vi "CalcDialogPanelBounds.vi"(8 "error in (no error)":errorcluster, 9 "Height":i32, 10 "Width":i32, 11 "Montior":i32) -> (0 "error out":errorcluster, 3 "Front Panel Window:Panel Bounds":T1)   [LabVIEW 2018, in "LcWebView.lvclass"]
doc: "This utility will fit (resize and center) a VI (defined by the \"VI Ref\" input) about the all of the Front Panel object. It will add a border defined by border spacing in units of pixels. If no VI Reference is passed in, it will operate on the calling VI."
uses:
  LcWebView.lvclass
  <vilib>/Utility/miscctls.llb/LVRectTypeDef.ctl
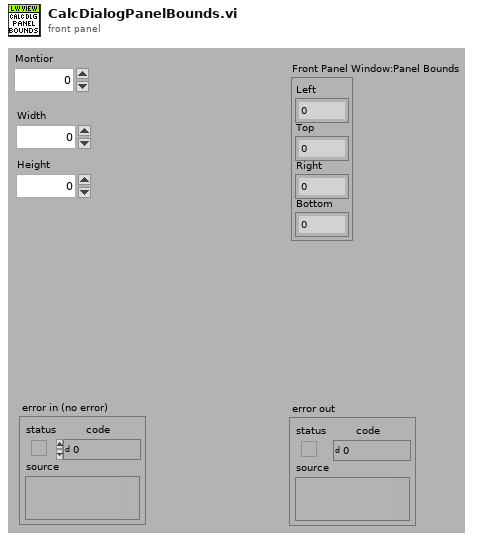
[diagram p1: front panel]
types:
  T1 = typedef "LVRectTypeDef.ctl" = cluster{"Left":i16, "Top":i16, "Right":i16, "Bottom":i16}
  T2 = typedef "LVAllMonitorsDisplayTypeDef.ctl" = cluster{"Bounds":cluster{"Left":i16, "Top":i16, "Right":i16, "Bottom":i16}, "Depth":i16}[]
  T3 = cluster{"Bounds":cluster{"Left":i16, "Top":i16, "Right":i16, "Bottom":i16}, "Depth":i16}
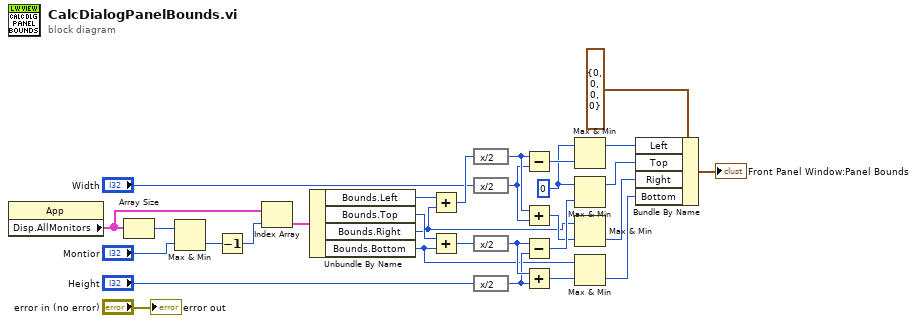
[diagram p0: block diagram]
diagram:
  w9 = 0 ("x")
  n1 = property class="App"() -> ("Disp.AllMonitors"=w13:T2)  [unwired: 2 in, 2 out]
  n2 = Array Size(array=w13) -> (size(s)=w12:i32)
  n3 = Max & Min(x=w12, y="Montior") -> (min(x,y)=w10:i32)  [unwired: 1 out]
  n4 = Decrement(x=w10) -> (x-1=w14:i32)
  n5 = Index Array(array=w13, index=w14) -> (element=w28:T3)
  n6 = Unbundle By Name(w28) -> ("Bounds.Left"=w27:i16, "Bounds.Top"=w24:i16, "Bounds.Right"=w2:i16, "Bounds.Bottom"=w1:i16)
  n7 = Add(x=w27, y=w2) -> (x+y=w26:i16)
  n8 = Add(x=w24, y=w1) -> (x+y=w25:i16)
  n9 = expression code="x/2"(w26) -> (w20:i16)
  n10 = expression code="x/2"("Width") -> (w19:i32)
  n11 = expression code="x/2"(w25) -> (w17:i16)
  n12 = expression code="x/2"("Height") -> (w16:i32)
  n13 = Subtract(x=w20, y=w19) -> (x-y=w18:i32)
  n14 = Add(x=w20, y=w19) -> (x+y=w6:i32)
  n15 = Subtract(x=w17, y=w16) -> (x-y=w15:i32)
  n16 = Add(x=w17, y=w16) -> (x+y=w4:i32)
  n17 = Max & Min(x=w9, y=w18) -> (max(x,y)=w8:i32)  [unwired: 1 out]
  n18 = Max & Min(x=w9, y=w15) -> (max(x,y)=w7:i32)  [unwired: 1 out]
  n19 = Max & Min(x=w2, y=w6) -> (min(x,y)=w5:i32)  [unwired: 1 out]
  n20 = Max & Min(x=w1, y=w4) -> (min(x,y)=w3:i32)  [unwired: 1 out]
  n21 = Bundle By Name(cluster=T1 {"Left"=0, "Top"=0, "Right"=0, "Bottom"=0} ("input cluster"), "Left"=w8, "Top"=w7, "Right"=w5, "Bottom"=w3) -> (→"Front Panel Window:Panel Bounds":T1)
  "error out" <- "error in (no error)"
